vi "Do.vi"(8 "error in":errorcluster, 10 "Actor in":refnum<class "Actor.lvclass">, 11 "Save Data MSG":refnum<class "Save Data MSG.lvclass">) -> (0 "error out":errorcluster, 2 "Actor out":refnum<class "Actor.lvclass">)   [LabVIEW 2017, in "Controller.lvlib" / "Save Data MSG.lvclass"]
doc: "(<B>Filename</B>: Actor Framework.lvlib:Message.lvclass:Do.vi)\n\nDefines what a message does when it is received by an actor. Generally, a message instructs an actor to invoke one of its methods. By default, this method does nothing. A child class must override it to define behavior. Create a child class by using the Actor Framework Message Maker dialog box."
uses:
  Save Data MSG.lvclass
  <vilib>/ActorFramework/Actor/Actor.lvclass
  File Actor/Messages/To/Save/Change File Writing State MSG.lvclass
  C:/Program Files (x86)/National Instruments/LabVIEW 2017/vi.lib/ActorFramework/Message/Message.lvclass
  gController.lvclass
  C:/Program Files (x86)/National Instruments/LabVIEW 2017/vi.lib/MSR Consulting, LLC/General Reuse/SuperActor/SuperActor.lvclass
  C:/Program Files (x86)/National Instruments/LabVIEW 2017/vi.lib/ActorFramework/Actor/Actor.lvclass
  <vilib>/ActorFramework/Message Enqueuer/Message Enqueuer.lvclass
  <vilib>/MSR Consulting, LLC/General Reuse/SuperActor/SuperActor.lvclass/SuperActor.ctl
  Save Data MSG.lvclass/Save Data MSG.ctl
  File Actor/Messages/To/Save/Change File Writing State MSG.lvclass/Change File Writing State MSG.ctl
  <vilib>/ActorFramework/Message Enqueuer/Message Enqueuer.lvclass/Message Enqueuer.ctl
  File Actor/Messages/To/Save/Write Save_.vi
  <vilib>/MSR Consulting, LLC/General Reuse/SuperActor/Read CVT Session.vi
  <vilib>/MSR Consulting, LLC/General Reuse/SuperActor/Read EnqueuerMap.vi
  <vilib>/MSR Consulting, LLC/General Reuse/SuperActor/Read Log Session.vi
  <vilib>/ActorFramework/Message Priority Queue/Priority Enqueue.vi
  <vilib>/MSR Consulting, LLC/General Reuse/Session APIs/_Session Fwk/Session - Root.lvclass
  <vilib>/MSR Consulting, LLC/General Reuse/Session APIs/CVT/CVT.lvclass
  <vilib>/MSR Consulting, LLC/General Reuse/Session APIs/Session Log/System Log.lvclass
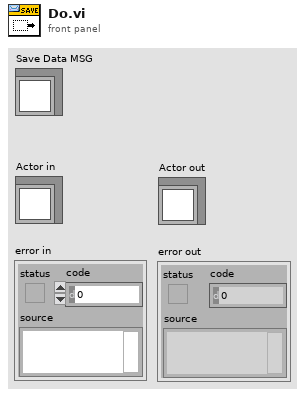
[diagram p1: front panel]
types:
  T1 = typedef "Session - Root.lvclass/Session Handle.ctl" = refnum<data-value>
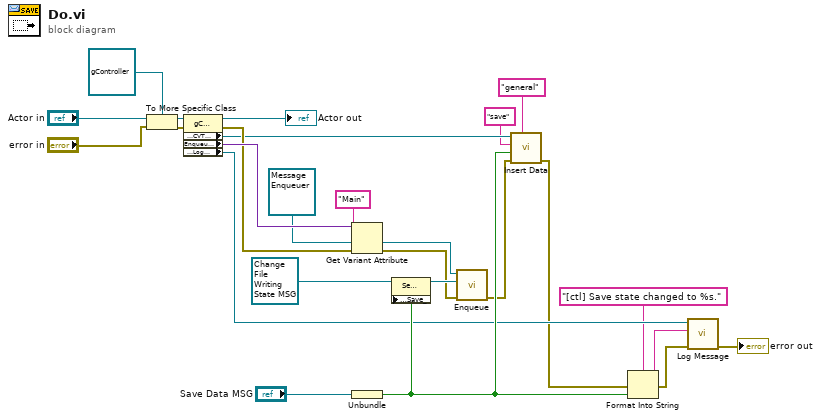
[diagram p0: block diagram]
diagram:
  n1 = To More Specific Class(target class=refnum<class "gController.lvclass"> refnum ("Controller.lvlib:gController"), reference="Actor in", error in="error in") -> (specific class reference=w24:refnum<class "gController.lvclass">, error out=w19:errorcluster)
  n2 = property class="gController"(reference=w24, error in=w19) -> (reference out=→"Actor out":refnum<class "gController.lvclass">, error out=w18:errorcluster, "Accessors:CVT Session"=w12:T1, "EnqueuerMap"=w23:variant, "Accessors:Log Session"=w8:T1)
  n3 = Get Variant Attribute(Variant=w23, name="Main", default value (empty Variant)=refnum<class "Message Enqueuer.lvclass"> refnum ("Self Enqueuer"), error in=w18) -> (value=w14:refnum<class "Message Enqueuer.lvclass">, error out=w7:errorcluster)  [unwired: 2 out]
  n4 = Unbundle("Save Data MSG") -> (w9:bool)
  n5 = property class="Set File Save State"(reference=refnum<class "Change File Writing State MSG.lvclass"> refnum ("File Library.lvlib:Set File Save State"), "Accessors:Save_"=w9) -> (reference out=w15:refnum<class "Change File Writing State MSG.lvclass">)  [unwired: 1 in, 1 out]
  n6 = call <vilib>:"Enqueue.vi"("error in (no error)"=w7, "Message"=w15, "Message Enqueuer in"=w14) -> ("error out"=w6:errorcluster)  [unwired: 7 in, 1 out]
  n7 = call <vilib>:"Insert Data.vi"("Group"="general", "error in"=w6, "Data"=w9, "tag"="save", "CVT Session In"=w12) -> ("error out"=w5:errorcluster)  [unwired: 5 in, 1 out]
  n8 = Format Into String(format string="[ctl] Save state changed to %s.", error in=w5, w9) -> (resulting string=w1:string, error out=w4:errorcluster)  [unwired: 1 in]
  n9 = call <vilib>:"Log Message.vi"("error in"=w4, "MSG In"=w1, "session in"=w8) -> ("error out"=→"error out":errorcluster)  [unwired: 7 in, 1 out]
